vi "3-temp1.vi"(3 "this":i32, 4 "button":i32, 5 "shift in":bool, 6 "settings in":T1={"Auto1"=TRUE, "Auto2"=TRUE, "Rel1"=TRUE, "Rel2"=TRUE, "Filt1"=TRUE, "Filt2"=TRUE, "Rate"=enum."Med", "Range1"=enum."10mV", "Range2"=enum."100mV", "Filt3"=TRUE, "Filt4"=TRUE, "Rel temp"=TRUE, "Analog1"=FALSE, "Analog2"=FALSE, "Analog temp"=FALSE, "Digital1"=TRUE, "Digital2"=TRUE, "Digital temp "=TRUE, "Window1"=enum."0,01%", "Window2"=enum."0,01%", "Window temp"=enum."0,01%", "RDGS1"="010", "RDGS2"="010", "RDGS temp"="010", "Type_type1"=TRUE, "Type_type2"=TRUE, "Type_type temp"=TRUE, "LSync"=FALSE, "Unit"=enum."C", "Sens"=TRUE, "Type tcoupl"=enum."J", "Junc"=TRUE}) -> (0 "next state":i32, 1 "shift out":bool, 2 "settings out":T1)   [LabVIEW 2017]
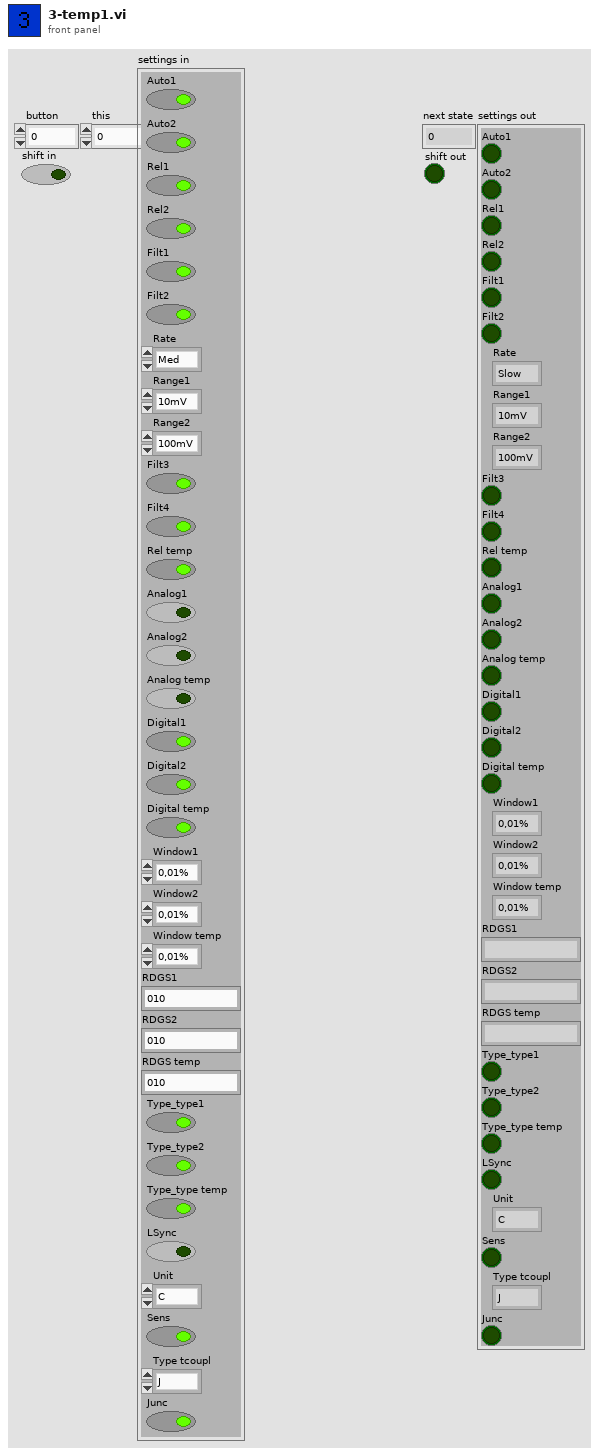
[diagram p1: front panel]
types:
  T1 = cluster{"Auto1":bool, "Auto2":bool, "Rel1":bool, "Rel2":bool, "Filt1":bool, "Filt2":bool, "Rate":enum16{"Slow", "Med", "Fast"}, "Range1":enum16{"10mV", "100mV", "1V", "10V", "100V"}, "Range2":enum16{"100mV", "1V", "10V"}, "Filt3":bool, "Filt4":bool, "Rel temp":bool, "Analog1":bool, "Analog2":bool, "Analog temp":bool, "Digital1":bool, "Digital2":bool, "Digital temp ":bool, "Window1":enum16{"0,01%", "0,1%", "1%", "10%", "None"}, "Window2":enum16{"0,01%", "0,1%", "1%", "10%", "None"}, "Window temp":enum16{"0,01%", "0,1%", "1%", "10%", "None"}, "RDGS1":string, "RDGS2":string, "RDGS temp":string, "Type_type1":bool, "Type_type2":bool, "Type_type temp":bool, "LSync":bool, "Unit":enum16{"C", "K", "F"}, "Sens":bool, "Type tcoupl":enum16{"J", "K", "T", "E", "R", "S", "B", "N"}, "Junc":bool}
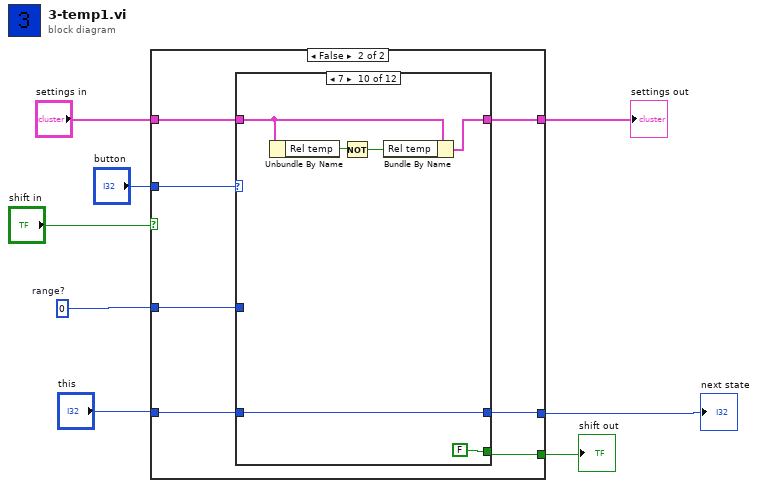
[diagram p0: block diagram]
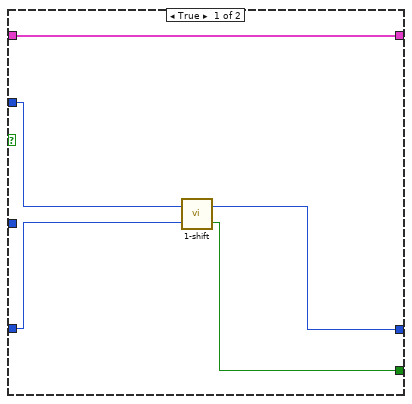
[diagram p2: hidden frame]
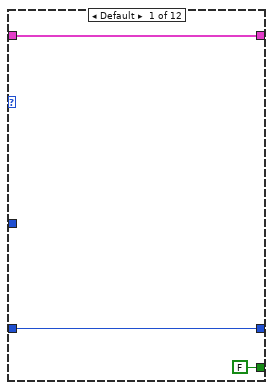
[diagram p3: hidden frame]
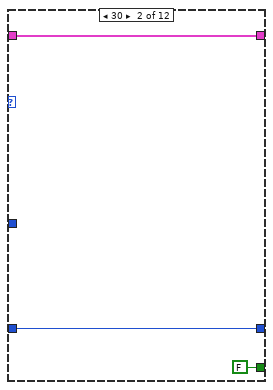
[diagram p4: hidden frame]
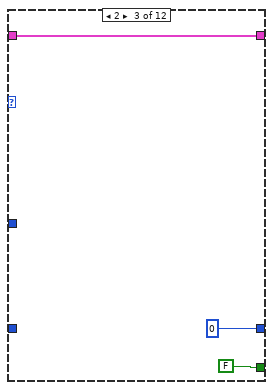
[diagram p5: hidden frame]
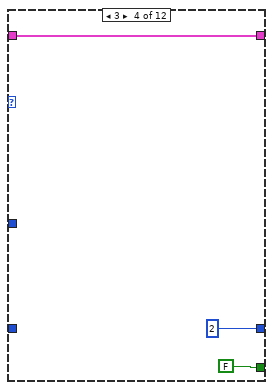
[diagram p6: hidden frame]
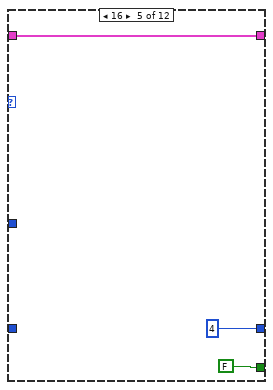
[diagram p7: hidden frame]
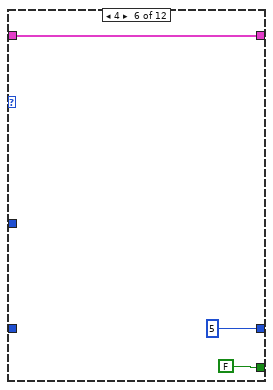
[diagram p8: hidden frame]
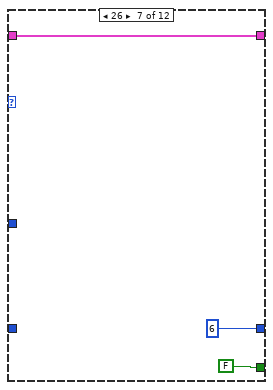
[diagram p9: hidden frame]
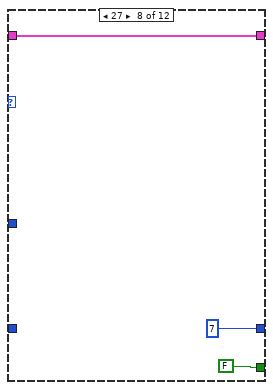
[diagram p10: hidden frame]
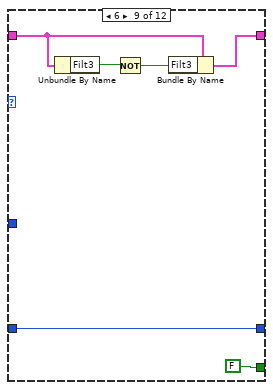
[diagram p11: hidden frame]
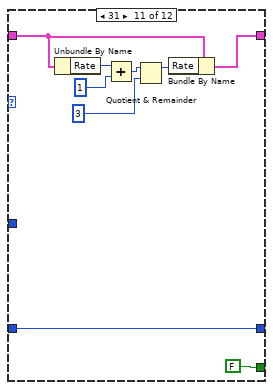
[diagram p12: hidden frame]
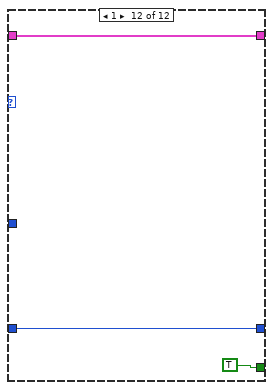
[diagram p13: hidden frame]
diagram:
  w1 = 0  # range?
  n1 = case shown="False" "shift in" {
    tunnel: "button" -> [w13 w20]
    tunnel: [w12 w19] -> w6
    tunnel: "this" -> [w11 w18]
    tunnel: [w9 w17] -> w4
    tunnel: "settings in" -> [w10 w16]
    tunnel: [w10 w15] -> w2
    tunnel: w1 -> [_ w14]
    frame True {
      n2 = call "1-shift.vi"("this"=w11, "button"=w13) -> ("shift"=w9:bool, "next state"=w12:i32)
    }
    frame False {
      n3 = case shown="7" w20 {
        tunnel: [w22 w25 0 2 4 5 6 7 w49 w55 w64 w68] -> w19
        tunnel: w18 -> [w22 w25 _ _ _ _ _ _ w49 w55 w64 w68]
        tunnel: [FALSE ("shift") FALSE ("shift") FALSE ("shift") FALSE ("shift") FALSE ("shift") FALSE ("shift") FALSE ("shift") FALSE ("shift") FALSE ("shift") FALSE ("shift") FALSE ("shift") TRUE ("shift")] -> w17
        tunnel: w16 -> [w23 w26 w27 w30 w33 w36 w39 w42 w46 w52 w63 w66]
        tunnel: [w23 w26 w27 w30 w33 w36 w39 w42 w45 w51 w62 w66] -> w15
        tunnel: w14 -> [_ _ _ _ _ _ _ _ _ _ _ _]
        frame Default {
        }
        frame 30 {
        }
        frame 2 {
        }
        frame 3 {
        }
        frame 16 {
        }
        frame 4 {
        }
        frame 26 {
        }
        frame 27 {
        }
        frame 6 {
          n4 = Unbundle By Name(w46) -> ("Filt3"=w48:bool)
          n5 = Not(x=w48) -> (.not. x?=w47:bool)
          n6 = Bundle By Name(cluster=w46, "Filt3"=w47) -> (w45:T1)
        }
        frame 7 {
          n7 = Unbundle By Name(w52) -> ("Rel temp"=w54:bool)
          n8 = Not(x=w54) -> (.not. x?=w53:bool)
          n9 = Bundle By Name(cluster=w52, "Rel temp"=w53) -> (w51:T1)
        }
        frame 31 {
          n10 = Unbundle By Name(w63) -> ("Rate"=w61:enum16{"Slow", "Med", "Fast"})
          n11 = Add(x=w61, y=1) -> (x+y=w59:i32)
          n12 = Quotient & Remainder(x=w59, y=3) -> (x-y*floor(x/y)=w58:i32)  [unwired: 1 out]
          n13 = Bundle By Name(cluster=w63, "Rate"=w58) -> (w62:T1)
        }
        frame 1 {
        }
      }
    }
  }
  "next state" <- w6
  "shift out" <- w4
  "settings out" <- w2
